vi "CRC Seeds.vi"   [LabVIEW 2014]
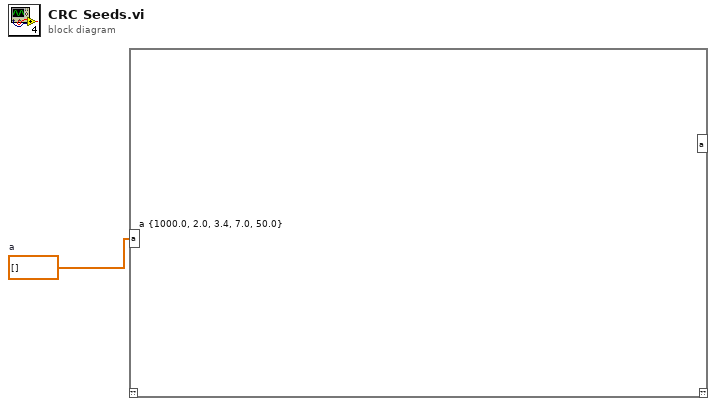
[diagram p0: block diagram]
diagram:
  w1 = dbl[] []  # a
  n1 = mathscript code="a {1000.0, 2.0, 3.4, 7.0, 50.0}"("a"=w1) -> ()  [unwired: 1 in, 2 out]
